vi "Digital_Bridge_3_kart.vi"() -> ()   [LabVIEW 2014] (continued)
                                n4674 = Index Array(array=w3706, index (row)=w3707, index (col)=w3704) -> (element=w3703:dbl)
                                n4675 = Replace Array Subset(array=w3706, new element=w3703, index (row)=w3707, index (col)=w3704) -> (w3705:dbl[][])
                                }
                                frame 6 {
                                n4676 = Index Array(array=w3709, index (row)=w3711, index (col)=w3710) -> (element=w3714:dbl)
                                n4677 = Multiply(x=w3714, y=2.0) -> (x*y=w3712:dbl)
                                n4678 = Replace Array Subset(array=w3709, new element=w3712, index (row)=w3711, index (col)=w3710) -> (w3708:dbl[][])
                                }
                                frame 7 {
                                n4679 = Index Array(array=w3716, index (row)=w3718, index (col)=w3717) -> (element=w3721:dbl)
                                n4680 = Multiply(x=w3721, y=2.0) -> (x*y=w3719:dbl)
                                n4681 = Replace Array Subset(array=w3716, new element=w3719, index (row)=w3718, index (col)=w3717) -> (w3715:dbl[][])
                                }
                                frame 8 {
                                n4682 = Index Array(array=w3725, index (row)=w3724, index (col)=w3723) -> (element=w3722:dbl)
                                n4683 = Replace Array Subset(array=w3725, new element=w3722, index (row)=w3724, index (col)=w3723) -> (w3726:dbl[][])
                                }
                                frame 9 {
                                n4684 = Index Array(array=w3730, index (row)=w3729, index (col)=w3728) -> (element=w3727:dbl)
                                n4685 = Replace Array Subset(array=w3730, new element=w3727, index (row)=w3729, index (col)=w3728) -> (w3731:dbl[][])
                                }
                                }
                                n4686 = local write "Denge Kosulu x1_x2"(w3675) -> ()
                                }
                                }
                                frame 5 {
                                n4687 = for {
                                N: 10 -> [_]
                                tunnel: w3732 -> [w3734]
                                i -> [w3737]
                                n4688 = local read "Denge Kosulu x1_x2"() -> (w3736:dbl[][])
                                n4689 = case shown="1" w3737 {
                                tunnel: w3737 -> [w3738 w3745 w3756 w3761 w3766 w3771 w3776 w3781 w3786 w3790]
                                tunnel: w3736 -> [w3739 w3747 w3755 w3760 w3765 w3770 w3774 w3779 w3787 w3791]
                                tunnel: [w3740 w3748 w3753 w3759 w3764 w3769 w3773 w3778 w3788 w3792] -> w3735
                                tunnel: w3734 -> [w3741 w3746 w3754 w3758 w3763 w3768 w3775 w3780 w3785 w3789]
                                frame 0, Default {
                                n4690 = Index Array(array=w3739, index (row)=w3738, index (col)=w3741) -> (element=w3744:dbl)
                                n4691 = Multiply(x=w3744, y=2.0) -> (x*y=w3742:dbl)
                                n4692 = Replace Array Subset(array=w3739, new element=w3742, index (row)=w3738, index (col)=w3741) -> (w3740:dbl[][])
                                }
                                frame 1 {
                                n4693 = Index Array(array=w3747, index (row)=w3745, index (col)=w3746) -> (element=w3751:dbl)
                                n4694 = Multiply(x=w3751, y=2.0) -> (x*y=w3749:dbl)
                                n4695 = Replace Array Subset(array=w3747, new element=w3749, index (row)=w3745, index (col)=w3746) -> (w3748:dbl[][])
                                }
                                frame 2 {
                                n4696 = Index Array(array=w3755, index (row)=w3756, index (col)=w3754) -> (element=w3752:dbl)
                                n4697 = Replace Array Subset(array=w3755, new element=w3752, index (row)=w3756, index (col)=w3754) -> (w3753:dbl[][])
                                }
                                frame 3 {
                                n4698 = Index Array(array=w3760, index (row)=w3761, index (col)=w3758) -> (element=w3757:dbl)
                                n4699 = Replace Array Subset(array=w3760, new element=w3757, index (row)=w3761, index (col)=w3758) -> (w3759:dbl[][])
                                }
                                frame 4 {
                                n4700 = Index Array(array=w3765, index (row)=w3766, index (col)=w3763) -> (element=w3762:dbl)
                                n4701 = Replace Array Subset(array=w3765, new element=w3762, index (row)=w3766, index (col)=w3763) -> (w3764:dbl[][])
                                }
                                frame 5 {
                                n4702 = Index Array(array=w3770, index (row)=w3771, index (col)=w3768) -> (element=w3767:dbl)
                                n4703 = Replace Array Subset(array=w3770, new element=w3767, index (row)=w3771, index (col)=w3768) -> (w3769:dbl[][])
                                }
                                frame 6 {
                                n4704 = Index Array(array=w3774, index (row)=w3776, index (col)=w3775) -> (element=w3772:dbl)
                                n4705 = Replace Array Subset(array=w3774, new element=w3772, index (row)=w3776, index (col)=w3775) -> (w3773:dbl[][])
                                }
                                frame 7 {
                                n4706 = Index Array(array=w3779, index (row)=w3781, index (col)=w3780) -> (element=w3777:dbl)
                                n4707 = Replace Array Subset(array=w3779, new element=w3777, index (row)=w3781, index (col)=w3780) -> (w3778:dbl[][])
                                }
                                frame 8 {
                                n4708 = Index Array(array=w3787, index (row)=w3786, index (col)=w3785) -> (element=w3784:dbl)
                                n4709 = Multiply(x=w3784, y=2.0) -> (x*y=w3782:dbl)
                                n4710 = Replace Array Subset(array=w3787, new element=w3782, index (row)=w3786, index (col)=w3785) -> (w3788:dbl[][])
                                }
                                frame 9 {
                                n4711 = Index Array(array=w3791, index (row)=w3790, index (col)=w3789) -> (element=w3795:dbl)
                                n4712 = Multiply(x=w3795, y=2.0) -> (x*y=w3793:dbl)
                                n4713 = Replace Array Subset(array=w3791, new element=w3793, index (row)=w3790, index (col)=w3789) -> (w3792:dbl[][])
                                }
                                }
                                n4714 = local write "Denge Kosulu x1_x2"(w3735) -> ()
                                }
                                }
                              }
                            }
                          }
                          frame #2 {
                            n4715 = for {
                              N: 5 -> [_]
                              tunnel: w3797 -> [w3800]
                              i -> [w3799]
                              n4716 = Increment(x=w3799) -> (x+1=w3798:i32)
                              n4717 = case shown="2" w3798 {
                                tunnel: w3800 -> [w3801 w3865 w3929 w3993 w4053]
                                frame 1 {
                                n4718 = for {
                                N: 10 -> [_]
                                tunnel: w3801 -> [w3803]
                                i -> [w3806]
                                n4719 = local read "Denge Kosulu y1_y2"() -> (w3805:dbl[][])
                                n4720 = case shown="0, Default" w3806 {
                                tunnel: w3806 -> [w3807 w3814 w3825 w3830 w3835 w3840 w3845 w3850 w3855 w3859]
                                tunnel: w3805 -> [w3808 w3816 w3824 w3829 w3834 w3839 w3843 w3848 w3856 w3860]
                                tunnel: [w3809 w3817 w3822 w3828 w3833 w3838 w3842 w3847 w3857 w3861] -> w3804
                                tunnel: w3803 -> [w3810 w3815 w3823 w3827 w3832 w3837 w3844 w3849 w3854 w3858]
                                frame 0, Default {
                                n4721 = Index Array(array=w3808, index (row)=w3807, index (col)=w3810) -> (element=w3813:dbl)
                                n4722 = Multiply(x=w3813, y=2.0) -> (x*y=w3811:dbl)
                                n4723 = Replace Array Subset(array=w3808, new element=w3811, index (row)=w3807, index (col)=w3810) -> (w3809:dbl[][])
                                }
                                frame 1 {
                                n4724 = Index Array(array=w3816, index (row)=w3814, index (col)=w3815) -> (element=w3820:dbl)
                                n4725 = Multiply(x=w3820, y=2.0) -> (x*y=w3818:dbl)
                                n4726 = Replace Array Subset(array=w3816, new element=w3818, index (row)=w3814, index (col)=w3815) -> (w3817:dbl[][])
                                }
                                frame 2 {
                                n4727 = Index Array(array=w3824, index (row)=w3825, index (col)=w3823) -> (element=w3821:dbl)
                                n4728 = Replace Array Subset(array=w3824, new element=w3821, index (row)=w3825, index (col)=w3823) -> (w3822:dbl[][])
                                }
                                frame 3 {
                                n4729 = Index Array(array=w3829, index (row)=w3830, index (col)=w3827) -> (element=w3826:dbl)
                                n4730 = Replace Array Subset(array=w3829, new element=w3826, index (row)=w3830, index (col)=w3827) -> (w3828:dbl[][])
                                }
                                frame 4 {
                                n4731 = Index Array(array=w3834, index (row)=w3835, index (col)=w3832) -> (element=w3831:dbl)
                                n4732 = Replace Array Subset(array=w3834, new element=w3831, index (row)=w3835, index (col)=w3832) -> (w3833:dbl[][])
                                }
                                frame 5 {
                                n4733 = Index Array(array=w3839, index (row)=w3840, index (col)=w3837) -> (element=w3836:dbl)
                                n4734 = Replace Array Subset(array=w3839, new element=w3836, index (row)=w3840, index (col)=w3837) -> (w3838:dbl[][])
                                }
                                frame 6 {
                                n4735 = Index Array(array=w3843, index (row)=w3845, index (col)=w3844) -> (element=w3841:dbl)
                                n4736 = Replace Array Subset(array=w3843, new element=w3841, index (row)=w3845, index (col)=w3844) -> (w3842:dbl[][])
                                }
                                frame 7 {
                                n4737 = Index Array(array=w3848, index (row)=w3850, index (col)=w3849) -> (element=w3846:dbl)
                                n4738 = Replace Array Subset(array=w3848, new element=w3846, index (row)=w3850, index (col)=w3849) -> (w3847:dbl[][])
                                }
                                frame 8 {
                                n4739 = Index Array(array=w3856, index (row)=w3855, index (col)=w3854) -> (element=w3853:dbl)
                                n4740 = Multiply(x=w3853, y=2.0) -> (x*y=w3851:dbl)
                                n4741 = Replace Array Subset(array=w3856, new element=w3851, index (row)=w3855, index (col)=w3854) -> (w3857:dbl[][])
                                }
                                frame 9 {
                                n4742 = Index Array(array=w3860, index (row)=w3859, index (col)=w3858) -> (element=w3864:dbl)
                                n4743 = Multiply(x=w3864, y=2.0) -> (x*y=w3862:dbl)
                                n4744 = Replace Array Subset(array=w3860, new element=w3862, index (row)=w3859, index (col)=w3858) -> (w3861:dbl[][])
                                }
                                }
                                n4745 = local write "Denge Kosulu y1_y2"(w3804) -> ()
                                }
                                }
                                frame 2 {
                                n4746 = for {
                                N: 10 -> [_]
                                tunnel: w3865 -> [w3867]
                                i -> [w3870]
                                n4747 = local read "Denge Kosulu y1_y2"() -> (w3869:dbl[][])
                                n4748 = case shown="0, Default" w3870 {
                                tunnel: w3870 -> [w3872 w3877 w3884 w3891 w3898 w3905 w3913 w3918 w3921 w3926]
                                tunnel: w3869 -> [w3873 w3879 w3883 w3890 w3897 w3904 w3911 w3916 w3922 w3927]
                                tunnel: [w3874 w3880 w3881 w3889 w3896 w3903 w3910 w3915 w3923 w3928] -> w3868
                                tunnel: w3867 -> [w3875 w3878 w3882 w3888 w3895 w3902 w3912 w3917 w3920 w3925]
                                frame 0, Default {
                                n4749 = Index Array(array=w3873, index (row)=w3872, index (col)=w3875) -> (element=w3871:dbl)
                                n4750 = Replace Array Subset(array=w3873, new element=w3871, index (row)=w3872, index (col)=w3875) -> (w3874:dbl[][])
                                }
                                frame 1 {
                                n4751 = Index Array(array=w3879, index (row)=w3877, index (col)=w3878) -> (element=w3876:dbl)
                                n4752 = Replace Array Subset(array=w3879, new element=w3876, index (row)=w3877, index (col)=w3878) -> (w3880:dbl[][])
                                }
                                frame 2 {
                                n4753 = Index Array(array=w3883, index (row)=w3884, index (col)=w3882) -> (element=w3887:dbl)
                                n4754 = Multiply(x=w3887, y=2.0) -> (x*y=w3885:dbl)
                                n4755 = Replace Array Subset(array=w3883, new element=w3885, index (row)=w3884, index (col)=w3882) -> (w3881:dbl[][])
                                }
                                frame 3 {
                                n4756 = Index Array(array=w3890, index (row)=w3891, index (col)=w3888) -> (element=w3894:dbl)
                                n4757 = Multiply(x=w3894, y=2.0) -> (x*y=w3892:dbl)
                                n4758 = Replace Array Subset(array=w3890, new element=w3892, index (row)=w3891, index (col)=w3888) -> (w3889:dbl[][])
                                }
                                frame 4 {
                                n4759 = Index Array(array=w3897, index (row)=w3898, index (col)=w3895) -> (element=w3901:dbl)
                                n4760 = Multiply(x=w3901, y=2.0) -> (x*y=w3899:dbl)
                                n4761 = Replace Array Subset(array=w3897, new element=w3899, index (row)=w3898, index (col)=w3895) -> (w3896:dbl[][])
                                }
                                frame 5 {
                                n4762 = Index Array(array=w3904, index (row)=w3905, index (col)=w3902) -> (element=w3908:dbl)
                                n4763 = Multiply(x=w3908, y=2.0) -> (x*y=w3906:dbl)
                                n4764 = Replace Array Subset(array=w3904, new element=w3906, index (row)=w3905, index (col)=w3902) -> (w3903:dbl[][])
                                }
                                frame 6 {
                                n4765 = Index Array(array=w3911, index (row)=w3913, index (col)=w3912) -> (element=w3909:dbl)
                                n4766 = Replace Array Subset(array=w3911, new element=w3909, index (row)=w3913, index (col)=w3912) -> (w3910:dbl[][])
                                }
                                frame 7 {
                                n4767 = Index Array(array=w3916, index (row)=w3918, index (col)=w3917) -> (element=w3914:dbl)
                                n4768 = Replace Array Subset(array=w3916, new element=w3914, index (row)=w3918, index (col)=w3917) -> (w3915:dbl[][])
                                }
                                frame 8 {
                                n4769 = Index Array(array=w3922, index (row)=w3921, index (col)=w3920) -> (element=w3919:dbl)
                                n4770 = Replace Array Subset(array=w3922, new element=w3919, index (row)=w3921, index (col)=w3920) -> (w3923:dbl[][])
                                }
                                frame 9 {
                                n4771 = Index Array(array=w3927, index (row)=w3926, index (col)=w3925) -> (element=w3924:dbl)
                                n4772 = Replace Array Subset(array=w3927, new element=w3924, index (row)=w3926, index (col)=w3925) -> (w3928:dbl[][])
                                }
                                }
                                n4773 = local write "Denge Kosulu y1_y2"(w3868) -> ()
                                }
                                }
                                frame 3 {
                                n4774 = for {
                                N: 10 -> [_]
                                tunnel: w3929 -> [w3931]
                                i -> [w3934]
                                n4775 = local read "Denge Kosulu y1_y2"() -> (w3933:dbl[][])
                                n4776 = case shown="0, Default" w3934 {
                                tunnel: w3934 -> [w3936 w3941 w3948 w3955 w3962 w3969 w3977 w3982 w3985 w3990]
                                tunnel: w3933 -> [w3937 w3943 w3947 w3954 w3961 w3968 w3975 w3980 w3986 w3991]
                                tunnel: [w3938 w3944 w3945 w3953 w3960 w3967 w3974 w3979 w3987 w3992] -> w3932
                                tunnel: w3931 -> [w3939 w3942 w3946 w3952 w3959 w3966 w3976 w3981 w3984 w3989]
                                frame 0, Default {
                                n4777 = Index Array(array=w3937, index (row)=w3936, index (col)=w3939) -> (element=w3935:dbl)
                                n4778 = Replace Array Subset(array=w3937, new element=w3935, index (row)=w3936, index (col)=w3939) -> (w3938:dbl[][])
                                }
                                frame 1 {
                                n4779 = Index Array(array=w3943, index (row)=w3941, index (col)=w3942) -> (element=w3940:dbl)
                                n4780 = Replace Array Subset(array=w3943, new element=w3940, index (row)=w3941, index (col)=w3942) -> (w3944:dbl[][])
                                }
                                frame 2 {
                                n4781 = Index Array(array=w3947, index (row)=w3948, index (col)=w3946) -> (element=w3951:dbl)
                                n4782 = Multiply(x=w3951, y=2.0) -> (x*y=w3949:dbl)
                                n4783 = Replace Array Subset(array=w3947, new element=w3949, index (row)=w3948, index (col)=w3946) -> (w3945:dbl[][])
                                }
                                frame 3 {
                                n4784 = Index Array(array=w3954, index (row)=w3955, index (col)=w3952) -> (element=w3958:dbl)
                                n4785 = Multiply(x=w3958, y=2.0) -> (x*y=w3956:dbl)
                                n4786 = Replace Array Subset(array=w3954, new element=w3956, index (row)=w3955, index (col)=w3952) -> (w3953:dbl[][])
                                }
                                frame 4 {
                                n4787 = Index Array(array=w3961, index (row)=w3962, index (col)=w3959) -> (element=w3965:dbl)
                                n4788 = Multiply(x=w3965, y=2.0) -> (x*y=w3963:dbl)
                                n4789 = Replace Array Subset(array=w3961, new element=w3963, index (row)=w3962, index (col)=w3959) -> (w3960:dbl[][])
                                }
                                frame 5 {
                                n4790 = Index Array(array=w3968, index (row)=w3969, index (col)=w3966) -> (element=w3972:dbl)
                                n4791 = Multiply(x=w3972, y=2.0) -> (x*y=w3970:dbl)
                                n4792 = Replace Array Subset(array=w3968, new element=w3970, index (row)=w3969, index (col)=w3966) -> (w3967:dbl[][])
                                }
                                frame 6 {
                                n4793 = Index Array(array=w3975, index (row)=w3977, index (col)=w3976) -> (element=w3973:dbl)
                                n4794 = Replace Array Subset(array=w3975, new element=w3973, index (row)=w3977, index (col)=w3976) -> (w3974:dbl[][])
                                }
                                frame 7 {
                                n4795 = Index Array(array=w3980, index (row)=w3982, index (col)=w3981) -> (element=w3978:dbl)
                                n4796 = Replace Array Subset(array=w3980, new element=w3978, index (row)=w3982, index (col)=w3981) -> (w3979:dbl[][])
                                }
                                frame 8 {
                                n4797 = Index Array(array=w3986, index (row)=w3985, index (col)=w3984) -> (element=w3983:dbl)
                                n4798 = Replace Array Subset(array=w3986, new element=w3983, index (row)=w3985, index (col)=w3984) -> (w3987:dbl[][])
                                }
                                frame 9 {
                                n4799 = Index Array(array=w3991, index (row)=w3990, index (col)=w3989) -> (element=w3988:dbl)
                                n4800 = Replace Array Subset(array=w3991, new element=w3988, index (row)=w3990, index (col)=w3989) -> (w3992:dbl[][])
                                }
                                }
                                n4801 = local write "Denge Kosulu y1_y2"(w3932) -> ()
                                }
                                }
                                frame 4, Default {
                                n4802 = for {
                                N: 10 -> [_]
                                tunnel: w3993 -> [w3995]
                                i -> [w3998]
                                n4803 = local read "Denge Kosulu y1_y2"() -> (w3997:dbl[][])
                                n4804 = case shown="0, Default" w3998 {
                                tunnel: w3998 -> [w4000 w4005 w4013 w4018 w4023 w4028 w4032 w4039 w4045 w4050]
                                tunnel: w3997 -> [w4001 w4007 w4012 w4017 w4022 w4027 w4030 w4037 w4046 w4051]
                                tunnel: [w4002 w4008 w4010 w4016 w4021 w4026 w4029 w4036 w4047 w4052] -> w3996
                                tunnel: w3995 -> [w4003 w4006 w4011 w4015 w4020 w4025 w4031 w4038 w4044 w4049]
                                frame 0, Default {
                                n4805 = Index Array(array=w4001, index (row)=w4000, index (col)=w4003) -> (element=w3999:dbl)
                                n4806 = Replace Array Subset(array=w4001, new element=w3999, index (row)=w4000, index (col)=w4003) -> (w4002:dbl[][])
                                }
                                frame 1 {
                                n4807 = Index Array(array=w4007, index (row)=w4005, index (col)=w4006) -> (element=w4004:dbl)
                                n4808 = Replace Array Subset(array=w4007, new element=w4004, index (row)=w4005, index (col)=w4006) -> (w4008:dbl[][])
                                }
                                frame 2 {
                                n4809 = Index Array(array=w4012, index (row)=w4013, index (col)=w4011) -> (element=w4009:dbl)
                                n4810 = Replace Array Subset(array=w4012, new element=w4009, index (row)=w4013, index (col)=w4011) -> (w4010:dbl[][])
                                }
                                frame 3 {
                                n4811 = Index Array(array=w4017, index (row)=w4018, index (col)=w4015) -> (element=w4014:dbl)
                                n4812 = Replace Array Subset(array=w4017, new element=w4014, index (row)=w4018, index (col)=w4015) -> (w4016:dbl[][])
                                }
                                frame 4 {
                                n4813 = Index Array(array=w4022, index (row)=w4023, index (col)=w4020) -> (element=w4019:dbl)
                                n4814 = Replace Array Subset(array=w4022, new element=w4019, index (row)=w4023, index (col)=w4020) -> (w4021:dbl[][])
                                }
                                frame 5 {
                                n4815 = Index Array(array=w4027, index (row)=w4028, index (col)=w4025) -> (element=w4024:dbl)
                                n4816 = Replace Array Subset(array=w4027, new element=w4024, index (row)=w4028, index (col)=w4025) -> (w4026:dbl[][])
                                }
                                frame 6 {
                                n4817 = Index Array(array=w4030, index (row)=w4032, index (col)=w4031) -> (element=w4035:dbl)
                                n4818 = Multiply(x=w4035, y=2.0) -> (x*y=w4033:dbl)
                                n4819 = Replace Array Subset(array=w4030, new element=w4033, index (row)=w4032, index (col)=w4031) -> (w4029:dbl[][])
                                }
                                frame 7 {
                                n4820 = Index Array(array=w4037, index (row)=w4039, index (col)=w4038) -> (element=w4042:dbl)
                                n4821 = Multiply(x=w4042, y=2.0) -> (x*y=w4040:dbl)
                                n4822 = Replace Array Subset(array=w4037, new element=w4040, index (row)=w4039, index (col)=w4038) -> (w4036:dbl[][])
                                }
                                frame 8 {
                                n4823 = Index Array(array=w4046, index (row)=w4045, index (col)=w4044) -> (element=w4043:dbl)
                                n4824 = Replace Array Subset(array=w4046, new element=w4043, index (row)=w4045, index (col)=w4044) -> (w4047:dbl[][])
                                }
                                frame 9 {
                                n4825 = Index Array(array=w4051, index (row)=w4050, index (col)=w4049) -> (element=w4048:dbl)
                                n4826 = Replace Array Subset(array=w4051, new element=w4048, index (row)=w4050, index (col)=w4049) -> (w4052:dbl[][])
                                }
                                }
                                n4827 = local write "Denge Kosulu y1_y2"(w3996) -> ()
                                }
                                }
                                frame 5 {
                                n4828 = for {
                                N: 10 -> [_]
                                tunnel: w4053 -> [w4055]
                                i -> [w4058]
                                n4829 = local read "Denge Kosulu y1_y2"() -> (w4057:dbl[][])
                                n4830 = case shown="0, Default" w4058 {
                                tunnel: w4058 -> [w4059 w4066 w4077 w4082 w4087 w4092 w4097 w4102 w4107 w4111]
                                tunnel: w4057 -> [w4060 w4068 w4076 w4081 w4086 w4091 w4095 w4100 w4108 w4112]
                                tunnel: [w4061 w4069 w4074 w4080 w4085 w4090 w4094 w4099 w4109 w4113] -> w4056
                                tunnel: w4055 -> [w4062 w4067 w4075 w4079 w4084 w4089 w4096 w4101 w4106 w4110]
                                frame 0, Default {
                                n4831 = Index Array(array=w4060, index (row)=w4059, index (col)=w4062) -> (element=w4065:dbl)
                                n4832 = Multiply(x=w4065, y=2.0) -> (x*y=w4063:dbl)
                                n4833 = Replace Array Subset(array=w4060, new element=w4063, index (row)=w4059, index (col)=w4062) -> (w4061:dbl[][])
                                }
                                frame 1 {
                                n4834 = Index Array(array=w4068, index (row)=w4066, index (col)=w4067) -> (element=w4072:dbl)
                                n4835 = Multiply(x=w4072, y=2.0) -> (x*y=w4070:dbl)
                                n4836 = Replace Array Subset(array=w4068, new element=w4070, index (row)=w4066, index (col)=w4067) -> (w4069:dbl[][])
                                }
                                frame 2 {
                                n4837 = Index Array(array=w4076, index (row)=w4077, index (col)=w4075) -> (element=w4073:dbl)
                                n4838 = Replace Array Subset(array=w4076, new element=w4073, index (row)=w4077, index (col)=w4075) -> (w4074:dbl[][])
                                }
                                frame 3 {
                                n4839 = Index Array(array=w4081, index (row)=w4082, index (col)=w4079) -> (element=w4078:dbl)
                                n4840 = Replace Array Subset(array=w4081, new element=w4078, index (row)=w4082, index (col)=w4079) -> (w4080:dbl[][])
                                }
                                frame 4 {
                                n4841 = Index Array(array=w4086, index (row)=w4087, index (col)=w4084) -> (element=w4083:dbl)
                                n4842 = Replace Array Subset(array=w4086, new element=w4083, index (row)=w4087, index (col)=w4084) -> (w4085:dbl[][])
                                }
                                frame 5 {
                                n4843 = Index Array(array=w4091, index (row)=w4092, index (col)=w4089) -> (element=w4088:dbl)
                                n4844 = Replace Array Subset(array=w4091, new element=w4088, index (row)=w4092, index (col)=w4089) -> (w4090:dbl[][])
                                }
                                frame 6 {
                                n4845 = Index Array(array=w4095, index (row)=w4097, index (col)=w4096) -> (element=w4093:dbl)
                                n4846 = Replace Array Subset(array=w4095, new element=w4093, index (row)=w4097, index (col)=w4096) -> (w4094:dbl[][])
                                }
                                frame 7 {
                                n4847 = Index Array(array=w4100, index (row)=w4102, index (col)=w4101) -> (element=w4098:dbl)
                                n4848 = Replace Array Subset(array=w4100, new element=w4098, index (row)=w4102, index (col)=w4101) -> (w4099:dbl[][])
                                }
                                frame 8 {
                                n4849 = Index Array(array=w4108, index (row)=w4107, index (col)=w4106) -> (element=w4105:dbl)
                                n4850 = Multiply(x=w4105, y=2.0) -> (x*y=w4103:dbl)
                                n4851 = Replace Array Subset(array=w4108, new element=w4103, index (row)=w4107, index (col)=w4106) -> (w4109:dbl[][])
                                }
                                frame 9 {
                                n4852 = Index Array(array=w4112, index (row)=w4111, index (col)=w4110) -> (element=w4116:dbl)
                                n4853 = Multiply(x=w4116, y=2.0) -> (x*y=w4114:dbl)
                                n4854 = Replace Array Subset(array=w4112, new element=w4114, index (row)=w4111, index (col)=w4110) -> (w4113:dbl[][])
                                }
                                }
                                n4855 = local write "Denge Kosulu y1_y2"(w4056) -> ()
                                }
                                }
                              }
                            }
                          }
                        }
                        n4856 = local read "frekans index"() -> (w3145:dbl)
                        n4857 = Equal?(x=w3145, y=0.0) -> (x = y?=w3143:bool)
                        n4858 = case shown="True" w3143 {
                          tunnel: [w3148 w3150] -> w3142
                          frame False {
                            n4859 = local read "frekans index"() -> (w3149:dbl)
                            n4860 = Decrement(x=w3149) -> (x-1=w3148:dbl)
                          }
                          frame True {
                            n4861 = local read "Frekanslar"() -> (w3152:dbl[])
                            n4862 = Array Size(array=w3152) -> (size(s)=w3153:i32)
                            n4863 = Decrement(x=w3153) -> (x-1=w3151:i32)
                            n4864 = To Double Precision Float(number=w3151) -> (double precision float=w3150:dbl)
                          }
                        }
                      }
                    }
                  }
                }
                n4865 = local read "count meas"() -> (w2069:u16)
                n4866 = local read "frekans index"() -> (w2068:dbl)
                n4867 = local read "control hz array"() -> (w2063:dbl[][])
                n4868 = Greater?(x=w2069, y=u16 8) -> (0:w2059:bool)
                n4869 = Equal?(x=w2068, y=0.0) -> (x = y?=w2066:bool)
                n4870 = case shown="True" w2066 {
                  tunnel: [w2075 w2077] -> w2056
                  frame False {
                    n4871 = local read "frekans index"() -> (w2076:dbl)
                    n4872 = Decrement(x=w2076) -> (x-1=w2075:dbl)
                  }
                  frame True {
                    n4873 = local read "Frekanslar"() -> (w2079:dbl[])
                    n4874 = Array Size(array=w2079) -> (size(s)=w2080:i32)
                    n4875 = Decrement(x=w2080) -> (x-1=w2078:i32)
                    n4876 = To Double Precision Float(number=w2078) -> (double precision float=w2077:dbl)
                  }
                }
                n4877 = call "change2d.vi"("reset(default false)"=FALSE, "index (col)"=w2056, "index (row)"=3, "read/write(T/F)"=TRUE, "2D Array"=w2063) -> ("result count"=w2064:dbl)  [unwired: 5 in, 1 out]
                n4878 = Greater?(x=w2064, y=0.0) -> (0:w2058:bool)
                n4879 = Or(x=w2059, y=w2058) -> (x .or. y?=w2057:bool)
                n4880 = case shown="True" w2057 {
                  tunnel: w2056 -> [w2081 w2092]
                  frame False {
                    n4881 = for {
                      N: 51 -> [_]
                      tunnel: w2081 -> [w2083]
                      i -> [w2084]
                      n4882 = local read "input values"() -> (w2086:dbl[])
                      n4883 = local read "F Values Array"() -> (w2089:dbl[][])
                      n4884 = local read "Frekanslar"() -> (w2088:dbl[])
                      n4885 = control-ref of="Frekans Listbox"() -> (w2090:refnum<vi>)
                      n4886 = Index Array(array=w2086, index=w2084) -> (element=w2085:dbl)
                      n4887 = call "change f values.vi"("index (col)"=w2084, "new element"=w2085, "frekans index"=w2083, "Frekanslar"=w2088, "F Values Array"=w2089, "LstBox Refnum"=w2090) -> ("output array"=w2087:dbl[][])  [unwired: 5 in]
                      n4888 = local write "F Values Array"(w2087) -> ()
                    }
                  }
                  frame True {
                    n4889 = for {
                      N: 51 -> [_]
                      tunnel: w2092 -> [w2160]
                      i -> [w2161]
                      n4890 = local read "input values 2"() -> (w2159:dbl[])
                      n4891 = for {
                        N: 5 -> [_]
                        shift-right: [w2167] -> w2157
                        shift-left: w2159 -> [w2172]
                        i -> [w2171]
                        n4892 = Add(x=4, y=w2171) -> (x+y=w2169:i32)
                        n4893 = Replace Array Subset(array=w2172, new element=0.0 ("new element/subarray"), index=w2169) -> (w2167:dbl[])
                      }
                      n4894 = local read "F Values Array"() -> (w2165:dbl[][])
                      n4895 = local read "Frekanslar"() -> (w2164:dbl[])
                      n4896 = control-ref of="Frekans Listbox"() -> (w2166:refnum<vi>)
                      n4897 = Index Array(array=w2157, index=w2161) -> (element=w2162:dbl)
                      n4898 = call "change f values.vi"("index (col)"=w2161, "new element"=w2162, "frekans index"=w2160, "Frekanslar"=w2164, "F Values Array"=w2165, "LstBox Refnum"=w2166) -> ("output array"=w2163:dbl[][])  [unwired: 5 in]
                      n4899 = local write "F Values Array"(w2163) -> ()
                    }
                    n4900 = for {
                      N: 5 -> [_]
                      tunnel: w2092 -> [w2096]
                      i -> [w2095]
                      n4901 = Increment(x=w2095) -> (x+1=w2094:i32)
                      n4902 = case shown="2" w2094 {
                        tunnel: w2096 -> [w2098 w2110 w2122 w2134 w2146]
                        frame 1 {
                          n4903 = local read "Frekanslar"() -> (w2102:dbl[])
                          n4904 = property on="Default Values Listbox" class="LstBox (strict)"() -> ("Item Names"=w2103:string[])  [unwired: 2 in, 2 out]
                          n4905 = Fract/Exp String To Number(string=w2103) -> (number=w2101:dbl[])  [unwired: 3 in, 1 out]
                          n4906 = Index Array(array=w2102, index=w2098) -> (element=w2099:dbl)
                          n4907 = Search 1D Array(1D array=w2101, element=w2099, start index (0)=0) -> (index of element=w2097:i32)
                          n4908 = local read "AD F/P Array"() -> (w2108:dbl[][])
                          n4909 = local read "Direnc 1 - Direnc 2"() -> (w2106:u32)
                          n4910 = Increment(x=w2106) -> (x+1=w2104:u32)
                          n4911 = Replace Array Subset(array=w2108, new element=0.0 ("new element/subarray"), index (row)=w2104, index (col)=w2097) -> (w2107:dbl[][])
                          n4912 = local write "AD F/P Array"(w2107) -> ()
                        }
                        frame 2 {
                          n4913 = local read "Frekanslar"() -> (w2114:dbl[])
                          n4914 = property on="Default Values Listbox" class="LstBox (strict)"() -> ("Item Names"=w2115:string[])  [unwired: 2 in, 2 out]
                          n4915 = Fract/Exp String To Number(string=w2115) -> (number=w2113:dbl[])  [unwired: 3 in, 1 out]
                          n4916 = Index Array(array=w2114, index=w2110) -> (element=w2111:dbl)
                          n4917 = local read "10R F/P Array"() -> (w2120:dbl[][])
                          n4918 = Search 1D Array(1D array=w2113, element=w2111, start index (0)=0) -> (index of element=w2109:i32)
                          n4919 = local read "Direnc 1 - Direnc 2"() -> (w2118:u32)
                          n4920 = Increment(x=w2118) -> (x+1=w2116:u32)
                          n4921 = Replace Array Subset(array=w2120, new element=0.0 ("new element/subarray"), index (row)=w2116, index (col)=w2109) -> (w2119:dbl[][])
                          n4922 = local write "10R F/P Array"(w2119) -> ()
                        }
                        frame 3 {
                          n4923 = local read "Frekanslar"() -> (w2126:dbl[])
                          n4924 = property on="Default Values Listbox" class="LstBox (strict)"() -> ("Item Names"=w2127:string[])  [unwired: 2 in, 2 out]
                          n4925 = Fract/Exp String To Number(string=w2127) -> (number=w2125:dbl[])  [unwired: 3 in, 1 out]
                          n4926 = Index Array(array=w2126, index=w2122) -> (element=w2123:dbl)
                          n4927 = Search 1D Array(1D array=w2125, element=w2123, start index (0)=0) -> (index of element=w2121:i32)
                          n4928 = local read "1R F/P Array"() -> (w2132:dbl[][])
                          n4929 = local read "Direnc 1 - Direnc 2"() -> (w2130:u32)
                          n4930 = Increment(x=w2130) -> (x+1=w2128:u32)
                          n4931 = Replace Array Subset(array=w2132, new element=0.0 ("new element/subarray"), index (row)=w2128, index (col)=w2121) -> (w2131:dbl[][])
                          n4932 = local write "1R F/P Array"(w2131) -> ()
                        }
                        frame 4, Default {
                          n4933 = local read "Frekanslar"() -> (w2138:dbl[])
                          n4934 = property on="Default Values Listbox" class="LstBox (strict)"() -> ("Item Names"=w2139:string[])  [unwired: 2 in, 2 out]
                          n4935 = Fract/Exp String To Number(string=w2139) -> (number=w2137:dbl[])  [unwired: 3 in, 1 out]
                          n4936 = Index Array(array=w2138, index=w2134) -> (element=w2135:dbl)
                          n4937 = Search 1D Array(1D array=w2137, element=w2135, start index (0)=0) -> (index of element=w2133:i32)
                          n4938 = local read "Wagner F/P Array"() -> (w2144:dbl[][])
                          n4939 = local read "Direnc 1 - Direnc 2"() -> (w2142:u32)
                          n4940 = Increment(x=w2142) -> (x+1=w2140:u32)
                          n4941 = Replace Array Subset(array=w2144, new element=0.0 ("new element/subarray"), index (row)=w2140, index (col)=w2133) -> (w2143:dbl[][])
                          n4942 = local write "Wagner F/P Array"(w2143) -> ()
                        }
                        frame 5 {
                          n4943 = local read "Frekanslar"() -> (w2150:dbl[])
                          n4944 = property on="Default Values Listbox" class="LstBox (strict)"() -> ("Item Names"=w2151:string[])  [unwired: 2 in, 2 out]
                          n4945 = Fract/Exp String To Number(string=w2151) -> (number=w2149:dbl[])  [unwired: 3 in, 1 out]
                          n4946 = Index Array(array=w2150, index=w2146) -> (element=w2147:dbl)
                          n4947 = Search 1D Array(1D array=w2149, element=w2147, start index (0)=0) -> (index of element=w2145:i32)
                          n4948 = local read "Kelvin F/P Array"() -> (w2156:dbl[][])
                          n4949 = local read "Direnc 1 - Direnc 2"() -> (w2154:u32)
                          n4950 = Increment(x=w2154) -> (x+1=w2152:u32)
                          n4951 = Replace Array Subset(array=w2156, new element=0.0 ("new element/subarray"), index (row)=w2152, index (col)=w2145) -> (w2155:dbl[][])
                          n4952 = local write "Kelvin F/P Array"(w2155) -> ()
                        }
                      }
                    }
                  }
                }
              }
              frame #5 {
                n4953 = local read "frekans index"() -> (w4154:dbl)
                n4954 = local read "control hz array"() -> (w4164:dbl[][])
                n4955 = local read "set"() -> (w4163:u16)
                n4956 = local read "control hz array"() -> (w4157:dbl[][])
                n4957 = local write "count meas"(u16 0 ("count meas")) -> ()
                n4958 = call "change2d.vi"("reset(default false)"=FALSE, "index (col)"=w4154, "index (row)"=3, "read/write(T/F)"=TRUE, "2D Array"=w4157) -> ("result count"=w4158:dbl)  [unwired: 5 in, 1 out]
                n4959 = local write "reset values"(FALSE ("reset values")) -> ()
                n4960 = call "check control hz array.vi"("count"=w4163, "control hz array"=w4164) -> ("logical AND"=w4162:bool)  [unwired: 9 in]
                n4961 = case shown="False" w4162 {
                  frame False {
                    n4962 = local write "BASLAT"(TRUE ("BASLAT")) -> ()
                  }
                  frame True {
                  }
                }
                n4963 = Greater?(x=w4158, y=0.0) -> (0:w4160:bool)
                n4964 = case shown="True" w4160 {
                  frame False {
                  }
                  frame True {
                    n4965 = local read "frekans index"() -> (w4166:dbl)
                    n4966 = local read "control hz array"() -> (w4169:dbl[][])
                    n4967 = call "change2d.vi"("reset(default false)"=TRUE, "index (col)"=w4166, "index (row)"=3, "read/write(T/F)"=FALSE, "2D Array"=w4169) -> ("2D Array Result"=w4170:dbl[][])  [unwired: 5 in, 1 out]
                    n4968 = local write "control hz array"(w4170) -> ()
                  }
                }
              }
            }
          }
        }
        n4969 = case shown="True" w614 {
          frame False {
          }
          frame True {
            n4970 = flat-sequence {
              frame #0 {
                n4971 = flat-sequence {
                  frame #0 {
                    "Other Array" <- dbl[] [] ("Other Array")
                    "Other Boolean Array" <- bool[] [] ("Other Boolean Array")
                    "input values" <- dbl[] [] ("values")
                    "F Values Array" <- dbl[][] [] ("F Values Array")
                  }
                  frame #1 {
                    n4972 = property on="Frekans Listbox" class="LstBox (strict)"() -> ("Item Names"=w1732:string[])  [unwired: 2 in, 2 out]
                    n4973 = Fract/Exp String To Number(string=w1732) -> (number=w1730:dbl[])  [unwired: 3 in, 1 out]
                    n4974 = Initialize Array(0.0 ("element"), 51 ("dimension size")) -> (w1718:dbl[])
                    n4975 = Array Size(array=w1730) -> (size(s)=w1729:i32)
                    n4976 = Initialize Array(0.0 ("element"), 10 ("dimension size")) -> (w1726:dbl[])
                    n4977 = Initialize Array(FALSE, 10 ("dimension size")) -> (w1727:bool[])
                    n4978 = Initialize Array(0.0 ("element"), w1729, 50 ("dimension size")) -> (w1721:dbl[][])
                    n4979 = local write "Other Array"(w1726) -> ()
                    n4980 = local write "Other Boolean Array"(w1727) -> ()
                    n4981 = local write "F Values Array"(w1721) -> ()
                    n4982 = local write "input values"(w1718) -> ()
                  }
                  frame #2 {
                    n4983 = flat-sequence {
                      frame #0 {
                        n4984 = local read "Frekans Listbox"() -> (w1733:i32[])
                        n4985 = local write "Default Values Listbox"(w1733) -> ()
                      }
                      frame #1 {
                        n4986 = property on="Frekans Listbox" class="LstBox (strict)"() -> ("Item Names"=w1735:string[])  [unwired: 2 in, 2 out]
                        n4987 = Array Size(array=w1735) -> (size(s)=w1734:i32)
                        n4988 = for {
                          N: w1734 -> [_]
                          i -> [w1737]
                          n4989 = property on="Default Values Listbox" class="LstBox (strict)"() -> ("Item Symbols"=w1739:i32[])  [unwired: 2 in, 2 out]
                          n4990 = Insert Into Array(array=w1739, index=w1737, new element=10 ("new element/subarray")) -> (w1738:i32[])
                          n4991 = property on="Default Values Listbox" class="LstBox (strict)"("Item Symbols"=w1738) -> ()  [unwired: 2 in, 2 out]
                        }
                      }
                      frame #2 {
                        n4992 = property on="Default Values Listbox" class="LstBox (strict)"() -> ("Item Names"=w1741:string[])  [unwired: 2 in, 2 out]
                        n4993 = Array Size(array=w1741) -> (size(s)=w1740:i32)
                        n4994 = for {
                          N: w1740 -> [_]
                          i -> [w1745]
                          n4995 = property on="Frekans Listbox" class="LstBox (strict)"() -> ("Item Symbols"=w1744:i32[])  [unwired: 2 in, 2 out]
                          n4996 = Insert Into Array(array=w1744, index=w1745, new element=10 ("new element/subarray")) -> (w1743:i32[])
                          n4997 = property on="Frekans Listbox" class="LstBox (strict)"("Item Symbols"=w1743) -> ()  [unwired: 2 in, 2 out]
                        }
                      }
                      frame #3 {
                        n4998 = property on="Default Values Listbox" class="LstBox (strict)"() -> ("Item Names"=w1746:string[])  [unwired: 2 in, 2 out]
                        n4999 = Array Size(array=w1746) -> (size(s)=w1747:i32)
                        n5000 = for {
                          N: w1747 -> [_]
                          tunnel: w1746 -> [w1748]
                          i -> [w1751]
                          n5001 = Fract/Exp String To Number(string=w1748) -> (number=w1749:dbl[])  [unwired: 3 in, 1 out]
                          n5002 = Index Array(array=w1749, index=w1751) -> (element=w1750:dbl)
                          n5003 = local read "F Values Array"() -> (w1754:dbl[][])
                          n5004 = Replace Array Subset(array=w1754, new element=w1750, index (row)=w1751, index (col)=0 ("disabled index (col)")) -> (w1753:dbl[][])
                          n5005 = local write "F Values Array"(w1753) -> ()
                        }
                      }
                    }
                  }
                }
                n5006 = flat-sequence {
                  frame #0 {
                    n5007 = property on="Direnc 1 - Direnc 2" class="Ring (strict)"() -> ("Strings []"=w1704:string[])  [unwired: 2 in, 2 out]
                    n5008 = property on="Frekans Listbox" class="LstBox (strict)"() -> ("Item Names"=w1707:string[])  [unwired: 2 in, 2 out]
                    n5009 = Array Size(array=w1707) -> (size(s)=w1705:i32)
                    n5010 = Array Size(array=w1704) -> (size(s)=w1706:i32)
                    n5011 = Fract/Exp String To Number(string=w1707) -> (number=w1708:dbl[])  [unwired: 3 in, 1 out]
                    n5012 = call "default_phase.vi"("dimension size y"=w1705, "dimension size x"=w1706, "frekanslar"=w1708) -> ("R/P Array"=→"Wagner F/P Array":dbl[][])  [unwired: 8 in]
                    n5013 = call "default_phase.vi"("dimension size y"=w1705, "dimension size x"=w1706, "frekanslar"=w1708) -> ("R/P Array"=→"1R F/P Array":dbl[][])  [unwired: 8 in]
                    n5014 = call "default_phase.vi"("dimension size y"=w1705, "dimension size x"=w1706, "frekanslar"=w1708) -> ("R/P Array"=→"10R F/P Array":dbl[][])  [unwired: 8 in]
                    n5015 = call "default_phase.vi"("dimension size y"=w1705, "dimension size x"=w1706, "frekanslar"=w1708) -> ("R/P Array"=→"AD F/P Array":dbl[][])  [unwired: 8 in]
                    n5016 = call "default_phase.vi"("dimension size y"=w1705, "dimension size x"=w1706, "frekanslar"=w1708) -> ("R/P Array"=→"Kelvin F/P Array":dbl[][])  [unwired: 8 in]
                  }
                }
                n5017 = flat-sequence {
                  frame #0 {
                    w1696 = FALSE ("Boolean 5")
                    w1697 = 0.0 ("amplitude 2/0")
                    w1698 = FALSE
                    w1699 = FALSE
                    n5018 = local write "PASS 10R"(w1699) -> ()
                    n5019 = local write "PASS 1R"(w1699) -> ()
                    n5020 = local write "PASS ANA D"(w1699) -> ()
                    n5021 = local write "PASS KELVIN"(w1699) -> ()
                    n5022 = local write "PASS WAGNER"(w1699) -> ()
                    n5023 = global write "DB_Global_4_kart-Test.vi" "amplitude 2/0"(w1697) -> ()
                    n5024 = global write "DB_Global_4_kart-Test.vi" "phase 2/ 0"(w1697) -> ()
                    n5025 = global write "DB_Global_4_kart-Test.vi" "amplitude 3/0"(w1697) -> ()
                    n5026 = global write "DB_Global_4_kart-Test.vi" "phase 3/0"(w1697) -> ()
                    n5027 = global write "DB_Global_4_kart-Test.vi" "amplitude 1/1"(w1697) -> ()
                    n5028 = global write "DB_Global_4_kart-Test.vi" "phase 1/1"(w1697) -> ()
                    n5029 = global write "DB_Global_4_kart-Test.vi" "amplitude 2/1"(w1697) -> ()
                    n5030 = global write "DB_Global_4_kart-Test.vi" "phase 2/1"(w1697) -> ()
                    n5031 = global write "DB_Global_4_kart-Test.vi" "amplitude 3/1"(w1697) -> ()
                    n5032 = global write "DB_Global_4_kart-Test.vi" "phase 3/1"(w1697) -> ()
                    n5033 = local write "KONTROL Y"(w1698) -> ()
                    n5034 = local write "KONTROL X"(w1698) -> ()
                    n5035 = local write "KONTROL Y 5"(w1698) -> ()
                    n5036 = local write "KONTROL X 5"(w1698) -> ()
                    n5037 = local write "KONTROL Y 3"(w1698) -> ()
                    n5038 = local write "KONTROL X 2"(w1698) -> ()
                    n5039 = local write "KONTROL Y 2"(w1698) -> ()
                    n5040 = local write "KONTROL X 3"(w1698) -> ()
                    n5041 = local write "KONTROL Y 4"(w1698) -> ()
                    n5042 = local write "KONTROL X 4"(w1698) -> ()
                    n5043 = local write "X"(w1698) -> ()
                    n5044 = local write "RANGE KONTROL X 5"(w1698) -> ()
                    n5045 = local write "Y"(w1698) -> ()
                    n5046 = local write "RANGE KONTROL X 2"(w1698) -> ()
                    n5047 = local write "X 2"(w1698) -> ()
                    n5048 = local write "RANGE KONTROL X 3"(w1698) -> ()
                    n5049 = local write "Y 2"(w1698) -> ()
                    n5050 = local write "RANGE KONTROL Y 5"(w1698) -> ()
                    n5051 = local write "X 3"(w1698) -> ()
                    n5052 = local write "RANGE KONTROL Y"(w1698) -> ()
                    n5053 = local write "Y 3"(w1698) -> ()
                    n5054 = local write "X1"(w1698) -> ()
                    n5055 = local write "IF ELSE X 5"(w1698) -> ()
                    n5056 = local write "Y1"(w1698) -> ()
                    n5057 = local write "IF ELSE Y 4"(w1698) -> ()
                    n5058 = local write "X1 2"(w1698) -> ()
